vi "mcc_etc_DIO_set.vi"(5 "degC_hi":dbl=45.0, 6 "error in":errorcluster, 7 "degC_low":dbl=5.0, 8 "degC_ch2":dbl, 9 "degC_ch1":dbl, 10 "input_line":refnum<k24>, 11 "output_line":refnum<k24>) -> (0 "DIO_control_status":bool, 1 "alarm":bool, 2 "input_line_out":refnum<k24>, 3 "output_line_out":refnum<k24>, 4 "error out":errorcluster)   [LabVIEW 2019]
uses:
  C:/Program Files/National Instruments/LabVIEW 2019/vi.lib/ULx/ULx_LV.dll
  Program Files/National Instruments/LabVIEW 2019/vi.lib/ULx/ULx_LV.dll
  <vilib>/ULx/Write.llb/ULx Write (Digital Bool 1Line 1Point).vi
  <vilib>/ULx/Read.llb/ULx Read (Digital Bool 1Line 1Point).vi
panel:
  out "alarm_read_back":bool
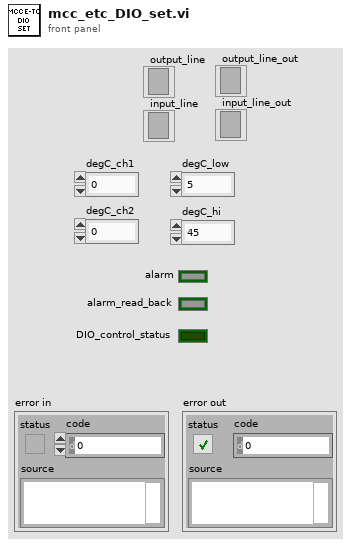
[diagram p1: front panel]
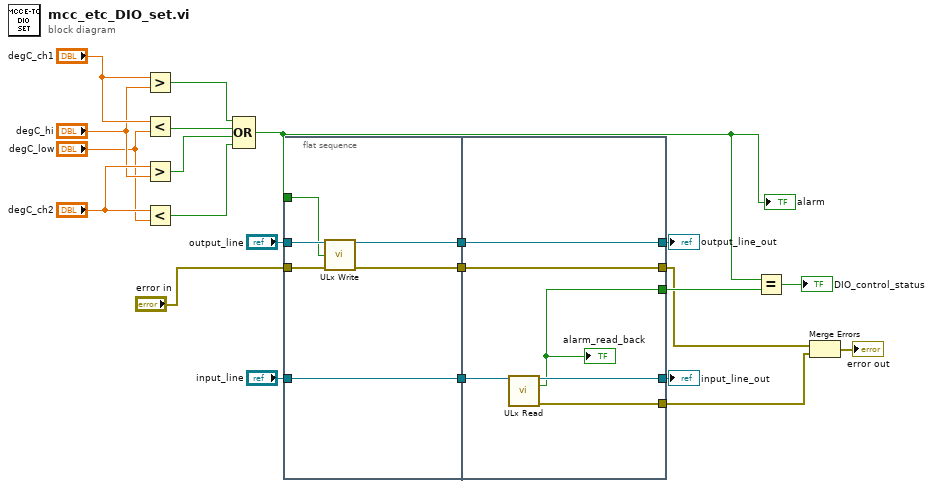
[diagram p0: block diagram]
diagram:
  n1 = Greater?(x="degC_ch1", y="degC_hi") -> (0:w11:bool)
  n2 = Less?(x="degC_ch1", y="degC_low") -> (x < y?=w10:bool)
  n3 = Greater?(x="degC_ch2", y="degC_hi") -> (0:w9:bool)
  n4 = Less?(x="degC_ch2", y="degC_low") -> (x < y?=w8:bool)
  n5 = Compound Arithmetic op=OR(w11, w10, w9, w8) -> (w7:bool)
  "alarm" <- w7
  n6 = flat-sequence {
    tunnel: "output_line" -> [w28]
    tunnel: w7 -> [w25]
    tunnel: [w27] -> w22
    tunnel: [w26] -> w21
    tunnel: "input_line" -> [w24]
    tunnel: [w24] -> w20
    tunnel: "error in" -> [w23]
    tunnel: [w33] -> w4
    tunnel: [w34] -> w17
    tunnel: w22 -> [w34]
    tunnel: w21 -> [w33]
    tunnel: w20 -> [w32]
    tunnel: [w31] -> w16
    tunnel: [w30] -> w3
    tunnel: [w29] -> w6
    frame #0 {
      n7 = call-poly <vilib>:"ULx Write.vi"("task in"=w28, "data"=w25, "error in"=w23) -> ("task out"=w27:refnum<k24>, "error out"=w26:errorcluster)  [unwired: 10 in, 1 out]
    }
    frame #1 {
      n8 = call-poly <vilib>:"ULx Read.vi"("task in"=w32) -> ("task out"=w31:refnum<k24>, "data"=w29:bool, "error out"=w30:errorcluster)  [unwired: 12 in]
      "alarm_read_back" <- w29
    }
  }
  n9 = Equal?(x=w7, y=w6) -> (x = y?=→"DIO_control_status":bool)
  n10 = Merge Errors(w4, w3) -> (→"error out":errorcluster)
  "output_line_out" <- w17
  "input_line_out" <- w16
